vi "WPI_AccelerometerADXL362_SPI_Close.vi"(8 "error in":errorcluster, 11 "AccelerometerDevRef":T1={"DevStatus"={"status"=FALSE, "code"=0, "source"=""}, "Scaling"={"Gain (VoltsPerG)"=0.0, "Center Voltage"=0.0}, "Analog Channels"={"X-Axis"=enum."Invalid", "Y-Axis"=enum."Invalid", "Z-Axis"=enum."Invalid"}, "I2C Bus"=enum."Invalid", "SPI Bus"=enum."Invalid", "Accel Range"=0, "ADXL Axes"={"X-Axis"=FALSE, "Y-Axis"=FALSE, "Z-Axis"=FALSE}, "Handle"=0, "Device Address"=0, "Accel Type"=enum."ADXL345 SPI"} {"Device Address" format="%.0x"; "Accel Range" items=["+/- 2 g", "+/- 4 g", "+/- 8 g", "+/- 16 g"]}) -> (0 "error out":errorcluster)   [LabVIEW 2017]
doc: "Closes the reference to the accelerometer you specify. Use this VI to close each accelerometer reference that you open with the Open VI.\n\nThis software is licensed. Open the labview\\readme\\WPI Robotics Library Open Source License.txt file for more information."
uses:
  <vilib>/Rock Robotics/WPI/Accelerometer/WPI_AccelerometerDevRef.ctl
  <vilib>/Rock Robotics/WPI/Accelerometer/WPI_AccelerometerScaling.ctl
  <vilib>/Rock Robotics/WPI/Accelerometer/WPI_AccelerometerAnalogChannels.ctl
  <vilib>/Rock Robotics/SystemInterfaces/AI/FPGA_AIChannel.ctl
  <vilib>/Rock Robotics/SystemInterfaces/i2clib/i2c_bus.ctl
  <vilib>/Rock Robotics/SystemInterfaces/spilib/spi_bus.ctl
  <vilib>/Rock Robotics/WPI/Accelerometer/ADXL345 Range.ctl
  <vilib>/Rock Robotics/WPI/Accelerometer/WPI_AccelerometerADXL345 Axes.ctl
  <vilib>/Rock Robotics/WPI/SPI/WPI_SPIDevRef.ctl
panel:
  # "ADXL"
  # "Analog"
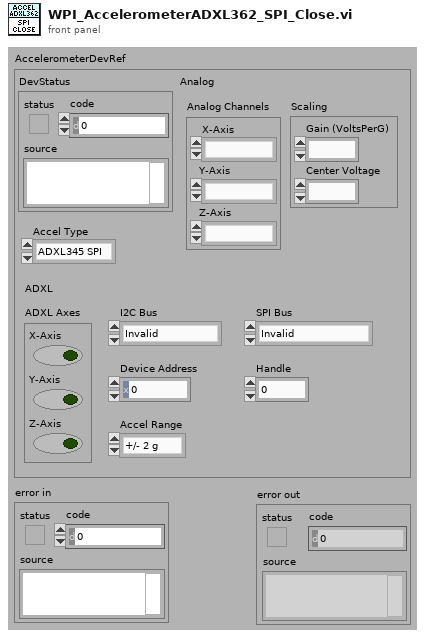
[diagram p1: front panel]
types:
  T1 = typedef "WPI_AccelerometerDevRef.ctl" = cluster{"DevStatus":errorcluster, "Scaling":T2, "Analog Channels":T3, "I2C Bus":T5, "SPI Bus":T6, "Accel Range":T7, "ADXL Axes":T8, "Handle":i32, "Device Address":u8, "Accel Type":enum16{"Analog", "ADXL345 I2C", "ADXL345 SPI", "Internal", "ADXL362 SPI"}}
  T2 = typedef "WPI_AccelerometerScaling.ctl" = cluster{"Gain (VoltsPerG)":dbl, "Center Voltage":dbl}
  T3 = typedef "WPI_AccelerometerAnalogChannels.ctl" = cluster{"X-Axis":T4, "Y-Axis":T4, "Z-Axis":T4}
  T4 = typedef "FPGA_AIChannel.ctl" = enum8{"AI 0", "AI 1", "AI 2", "AI 3", "AI MXP 0", "AI MXP 1", "AI MXP 2", "AI MXP 3", "Invalid"}
  T5 = typedef "i2c_bus.ctl" = enum16{"I2C On-Board", "I2C MXP", "Invalid"}
  T6 = typedef "spi_bus.ctl" = enum16{"SPI On-Board, CS0", "SPI On-Board, CS1", "SPI On-Board, CS2", "SPI On-Board, CS3", "SPI MXP", "Invalid"}
  T7 = typedef "ADXL345 Range.ctl" = u8
  T8 = typedef "WPI_AccelerometerADXL345 Axes.ctl" = cluster{"X-Axis":bool, "Y-Axis":bool, "Z-Axis":bool}
  T9 = typedef "WPI_SPIDevRef.ctl" = cluster{"DevStatus":errorcluster, "Handle":i32, "SPI Bus":T6}
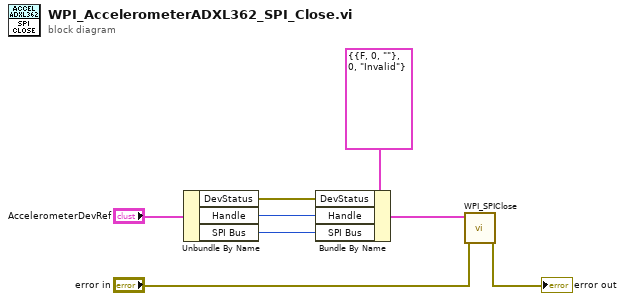
[diagram p0: block diagram]
diagram:
  n1 = Unbundle By Name("AccelerometerDevRef") -> ("DevStatus"=w7:errorcluster, "Handle"=w6:i32, "SPI Bus"=w5:T6)
  n2 = Bundle By Name(cluster=T9 {"DevStatus"={"status"=FALSE, "code"=0, "source"=""}, "Handle"=0, "SPI Bus"=enum."Invalid"} ("SPIDevRef"), "DevStatus"=w7, "Handle"=w6, "SPI Bus"=w5) -> (w2:T9)
  n3 = call <vilib>:"WPI_SPIClose.vi"("error in (no error)"="error in", "SPIDevRef"=w2) -> ("error out"=→"error out":errorcluster)  [unwired: 9 out]
